vi "get_total_number_of_pixels_per_cycle.vi"(8 "error in (no error)":errorcluster, 11 "TrajectoryAK101022Resonance in":refnum<class "TrajectoryAK101022Resonance.lvclass">) -> (0 "error out":errorcluster, 2 "total number of pixels per cycle":i32, 3 "TrajectoryAK101022Resonance out":refnum<class "TrajectoryAK101022Resonance.lvclass">)   [LabVIEW 2010, in "TrajectoryAK101022Resonance.lvclass"]
doc: "returns the total number of pixels of one complete scan cycle/repetition"
uses:
  TrajectoryAK101022Resonance.lvclass
  TrajectoryAK101022Resonance.lvclass/TrajectoryAK101022Resonance.ctl
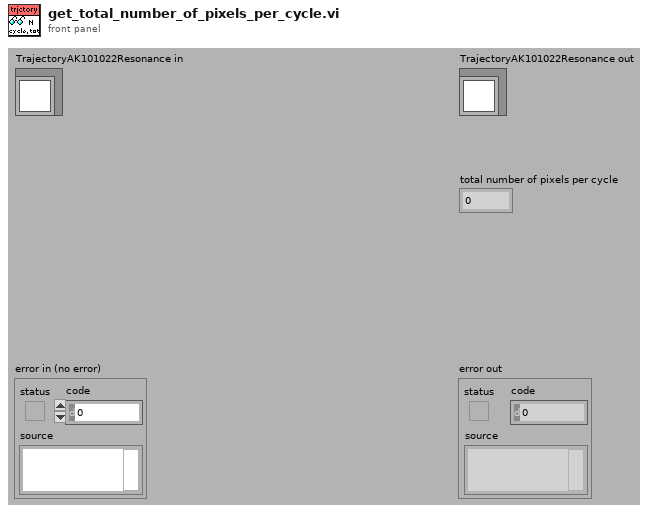
[diagram p1: front panel]
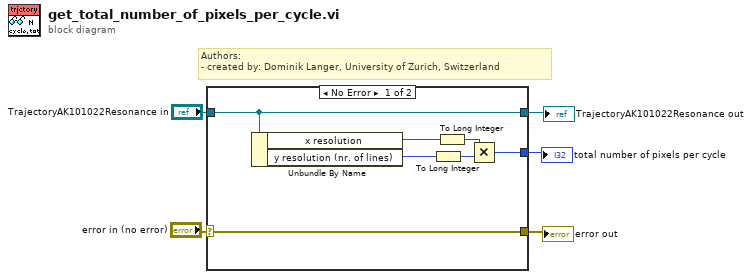
[diagram p0: block diagram]
diagram:
  # "Authors: \n- created by: Dominik Langer, University of Zurich, Switzerland"
  n1 = case shown="No Error" "error in (no error)" {
    selector: "error in (no error)" -> [w12 w13]
    tunnel: "TrajectoryAK101022Resonance in" -> [w11 w14]
    tunnel: [w12 w13] -> w3
    tunnel: [w11 w14] -> w2
    tunnel: [w10 _] -> w1
    frame No Error {
      n2 = Unbundle By Name(w11) -> ("x resolution"=w6:i32, "y resolution (nr. of lines)"=w7:i32)
      n3 = To Long Integer(number=w7) -> (32bit integer=w9:i32)
      n4 = To Long Integer(number=w6) -> (32bit integer=w8:i32)
      n5 = Multiply(x=w8, y=w9) -> (x*y=w10:i32)
    }
    frame Error {
    }
  }
  "error out" <- w3
  "TrajectoryAK101022Resonance out" <- w2
  "total number of pixels per cycle" <- w1
